vi "setTemperature__.vi"(8 "error in (no error)":errorcluster, 10 "temperature[°C]":i32, 11 "OvenController in":refnum<class "OvenController.lvclass">) -> (0 "error out":errorcluster, 3 "OvenController out":refnum<class "OvenController.lvclass">)   [LabVIEW 2023, in "AbstractFactory.lvlib" / "OvenController.lvclass"]
uses:
  OvenController.lvclass
  OvenController.lvclass/OvenController.ctl
  IConnection/IConnection.lvclass
  ICommandBuilder/ICommandBuilder.lvclass
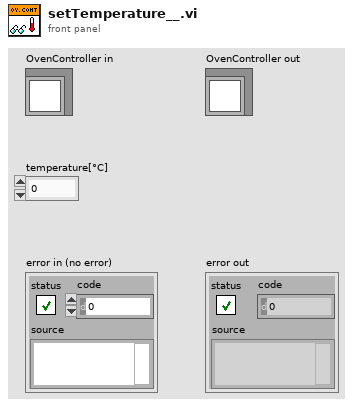
[diagram p1: front panel]
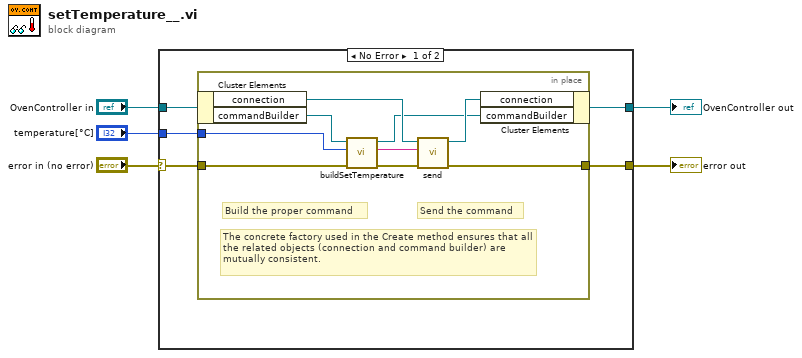
[diagram p0: block diagram]
diagram:
  n1 = case shown="No Error" "error in (no error)" {
    selector: "error in (no error)" -> [w8 w21]
    tunnel: [w7 w21] -> w4
    tunnel: [w10 w20] -> w2
    tunnel: "OvenController in" -> [w9 w20]
    tunnel: "temperature[°C]" -> [w6 _]
    frame No Error {
      n2 = in-place {
        in-place-border: w8 -> [w14]
        in-place-border: [w17] -> w7
        in-place-border: w6 -> [w12]
        # "The concrete factory used in the Create method ensures that all the related objects (connection and command builder) are mutually consistent."
        # "Send the command"
        # "Build the proper command"
        n3 = in-place-cluster #1(w9) -> ("connection"=w19:refnum<class "IConnection.lvclass">, "commandBuilder"=w16:refnum<class "ICommandBuilder.lvclass">)
        n4 = call-dynamic "buildSetTemperature.vi"("error in (no error)"=w14, "temperature[°C]"=w12, "ICommandBuilder in"=w16) -> ("error out"=w15:errorcluster, "message"=w11:string, "ICommandBuilder out"=w13:refnum<class "ICommandBuilder.lvclass">)  [unwired: 6 in]
        n5 = call-dynamic "send.vi"("error in (no error)"=w15, "message"=w11, "IConnection in"=w19) -> ("error out"=w17:errorcluster, "IConnection out"=w18:refnum<class "IConnection.lvclass">)  [unwired: 7 in]
        n6 = in-place-cluster #1("connection"=w18, "commandBuilder"=w13) -> (w10:refnum<class "OvenController.lvclass">)
      }
    }
    frame Error {
    }
  }
  "error out" <- w4
  "OvenController out" <- w2
